vi "Multi_Point_TraverseControl.vi"(0 "Mode":T2=enum."Read traverse position", 1 "Route Checking?":bool, 3 "Traverse Name":string, 5 "RollPitchYaw":dbl[](array[numeric]) caption="Model       Roll      Pitch       Yaw (deg)" format="%#.2f", 9 "Points to plot":dbl[][](array[numeric]) format="%.2f", 11 "Work in Tunnel Coordinates?":T1, 13 "Speed Factor":dbl=1.0 min=0.1 max=5.0 format="%.2f", 14 "Backlash Compensation?":bool=TRUE) -> (4 "Position Output XYZ":dbl[](array[numeric]) format="%.2f", 15 "Error String":string)   [LabVIEW 2014]
uses:
  Anemometry/Anemometry Sub Vis/Gen Trav/Trav_mode.ctl
  Anemometry/Anemometry Sub Vis/Controls/Tunnel_Coordinates.ctl
  Anemometry/Anemometry Sub Vis/Controls/Home.ctl
  ~subVIs/GenericDriveCommand.ctl
  ADAM Client/Sub VIs/ADAM Controls/Update_scan_value.ctl
  Anemometry/Anemometry Sub Vis/Globals/Trav_pos_global.vi
  Anemometry/Anemometry Sub Vis/Globals/Preference_global.vi
  ~subVIs/DriveConfigGlobal.vi
  Anemometry/Anemometry Sub Vis/Gen Trav/Route mapping/Route_mapping_global.vi
panel:
  out "Server copy Location":path
  out "Log File":path
  out "Achieved Pos In Eng units of all channels":dbl[](array[numeric]) format="%.2f"
  out "Pulses Positon all channels":dbl[](array[numeric])
  out "Counters Reset?":bool
  # "X                Y                   Z"
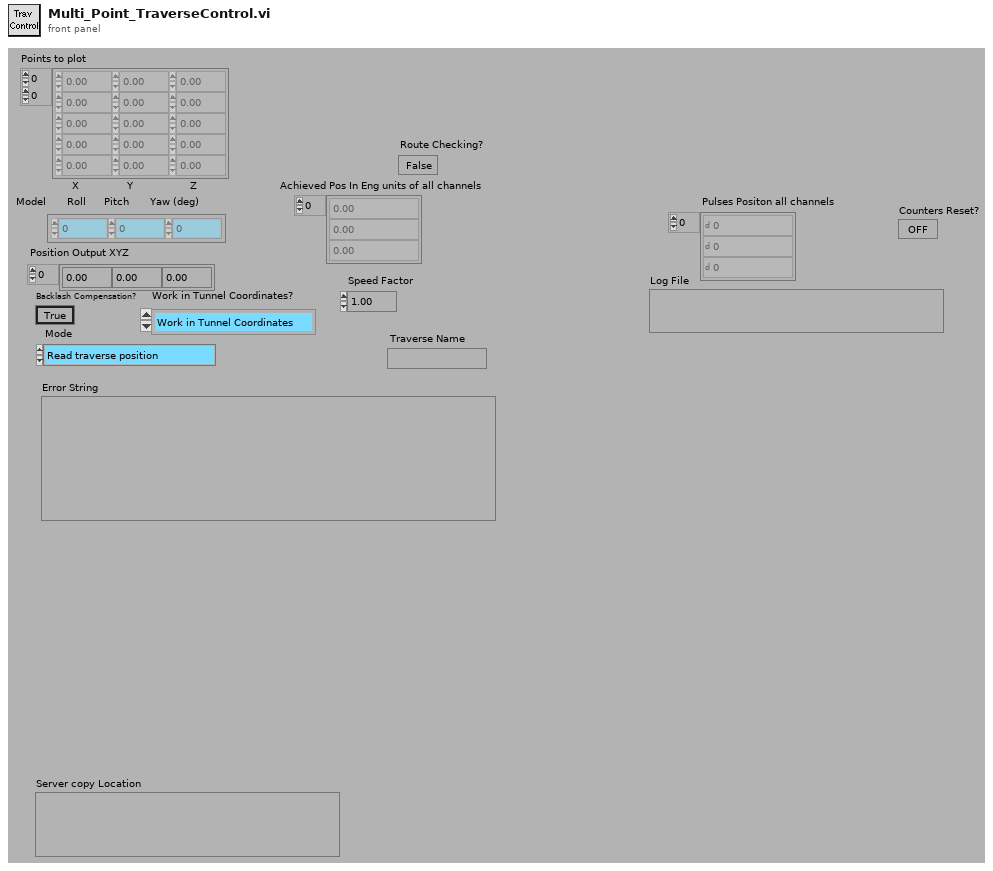
[diagram p1: front panel]
types:
  T1 = typedef "Tunnel_Coordinates.ctl" = enum16{"Work in Tunnel Coordinates", "Work in Model Coordinates"}
  T2 = typedef "Trav_mode.ctl" = enum16{"Move traverse", "Read traverse position", "Teach Position"}
  T3 = typedef "Home.ctl" = enum16{"Don't Home", "Home  +X", "Home  -X", "Home  +Y", "Home  -Y", "Home  +Z", "Home  -Z"}
  T4 = typedef "GenericDriveCommand.ctl" = string
  T5 = enum16{"To Traverse Coordinates", "To User Coordinates"}
  T6 = typedef "Update_scan_value.ctl" = cluster{"Channel Name":string, "New Value":dbl}
  T7 = typedef "AxisConfigCluster.ctl" = cluster{"Channel Properties":T8, "Static Drive Configuration":T9}
  T8 = typedef "DriveProperties.ctl" = cluster{"Channel Name":string, "Vel. Default":dbl, "Acc. Default":dbl, "Vel. Max":dbl, "Vel. Min":dbl, "Acc. Max":dbl, "Acc. Min":dbl, "Pulses/unit":dbl, "Address":u8, "Pulse Offset":i32, "Pos Tolerance":dbl, "Pulses/rev":dbl, "Backlash/Eng units":dbl, "Current Pos":dbl, "Ch Status":enum16{"Active", "Offline", "Simulate"}, "Port Name":string, "Axis Transform mode":string, "Metadata Ch Name":string, "Type":string}
  T9 = typedef "DriveStaticConfig.ctl" = cluster{"Correction Gain % (CG)":u16, "Dead Band (DB)":i32, "Dead Band Window (DW)":i32, "Encoder Resolution (ER)":i32, "Step Mode  (FSB)":u16, "Position Maintenance (FSC)":u16, "Stop on Stall (FSD)":u16, "Activate OP1 on stall (FSE)":u16, "Stop on Trigger 3 (FSF)":u16, "OP2 in Deadband (FSG)":u16, "Stall Detect (FSH)":u16, "Limit Disable (LD)":u16, "Motor Resolution (MR)":enum16{"200", "400", "1000", "2000", "4000", "5000", "10000", "12800", "18000", "20000", "21600", "25000", "25400", "25600", "36000", "50000", "278528", "425984", "507904", "614400", "655360", "819200", "1024000"}, "Limit Switch Sense (OSA)":u16, "Home Position (OSB)":u16, "Home Switch Sense (OSC)":u16, "Encoder Z for Home (OSD)":u16, "Reference edge of Home (OSH)":u16, "RS232 Echo Control (SSA)":u16, "Buffer at Limit (SSG)":u16, "Buffer at Stop (SSH)":u16, "Indexer Mode  (FSA)":u16, "Type":string, "ConfigString":string, "De Power Motor":enum16{"TRUE", "FALSE"}}
  T10 = typedef "Box_size.ctl" = cluster{"Max":dbl, "Min":dbl}[]
  T11 = typedef "Exclude_cluster.ctl" = cluster{"Sizes":T10, "Name":string, "Exclude Type":T12}
  T12 = typedef "Exclusion_type.ctl" = enum16{"Exclude completely", "Allow only vertical moves"}
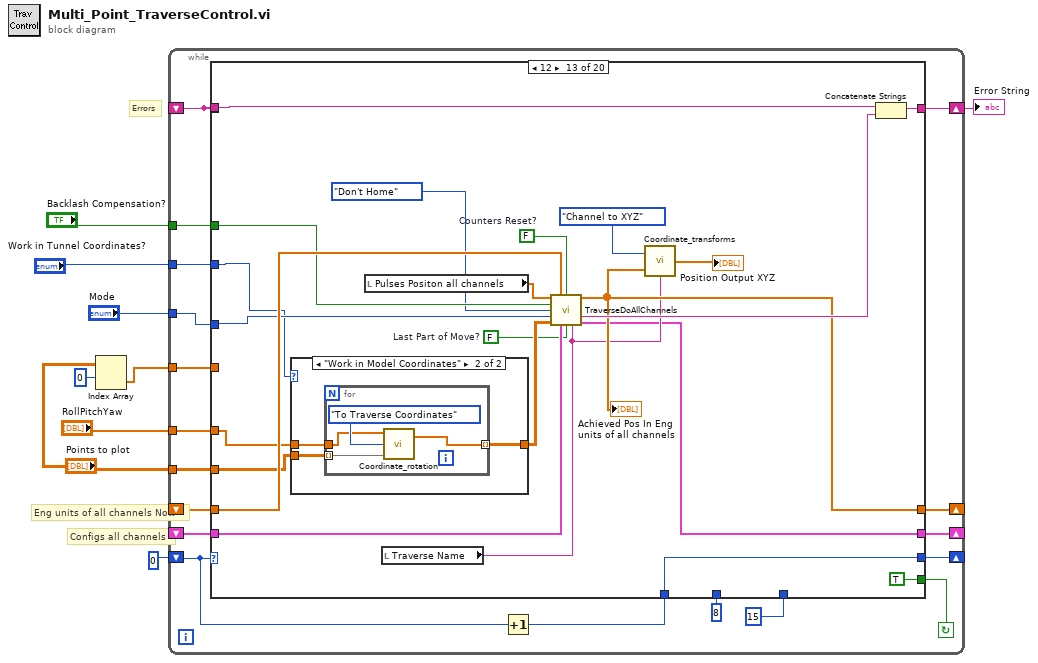
[diagram p0: block diagram]
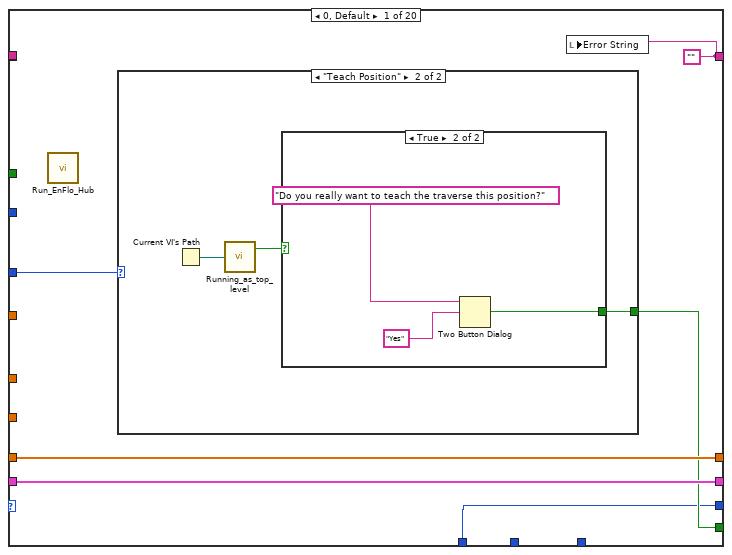
[diagram p2: hidden frame]
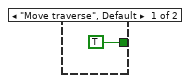
[diagram p3: hidden frame]
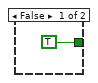
[diagram p4: hidden frame]
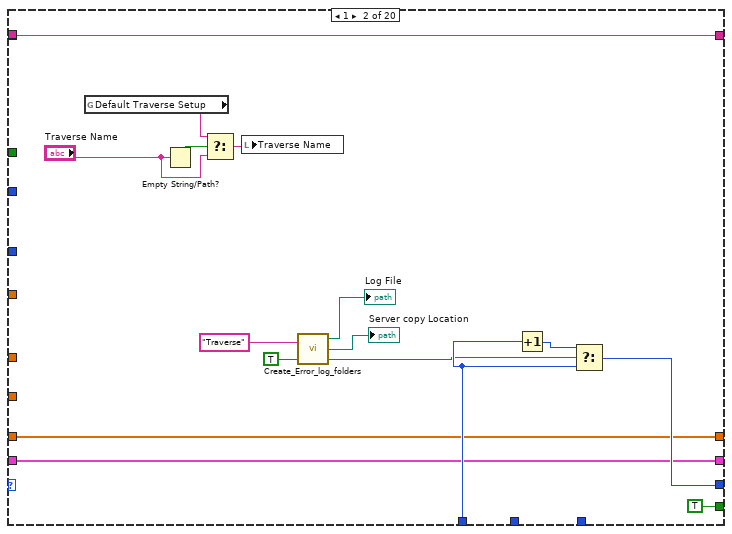
[diagram p5: hidden frame]
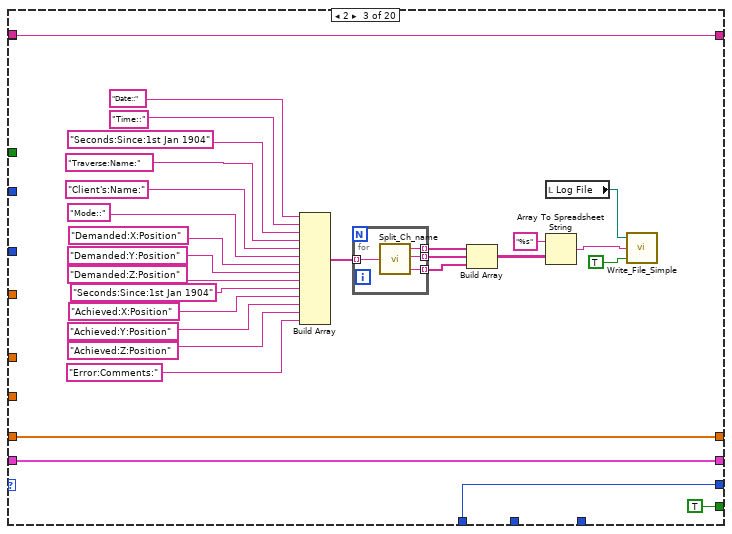
[diagram p6: hidden frame]
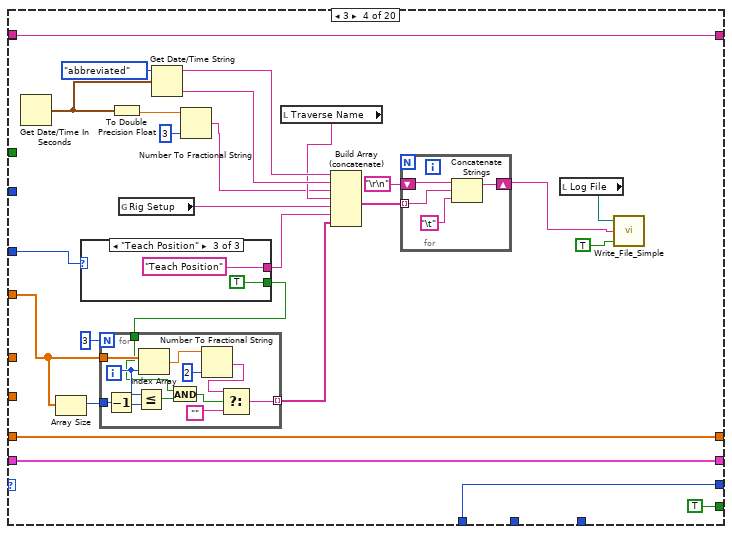
[diagram p7: hidden frame]
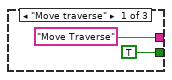
[diagram p8: hidden frame]
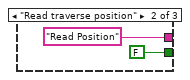
[diagram p9: hidden frame]
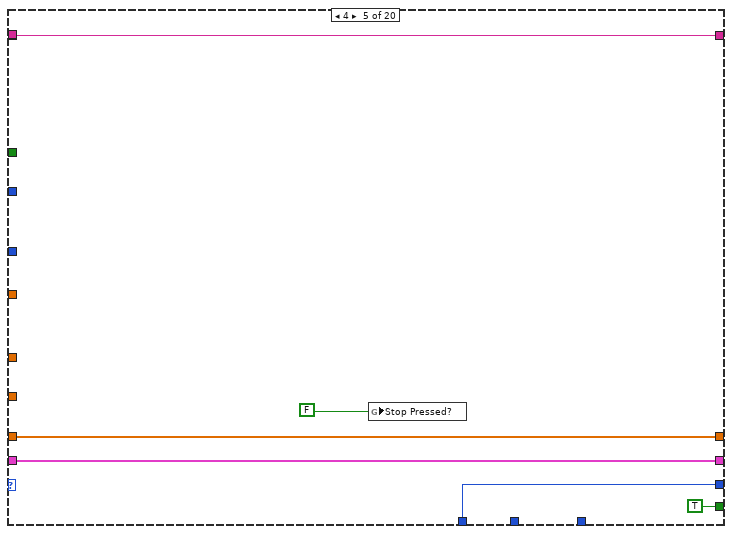
[diagram p10: hidden frame]
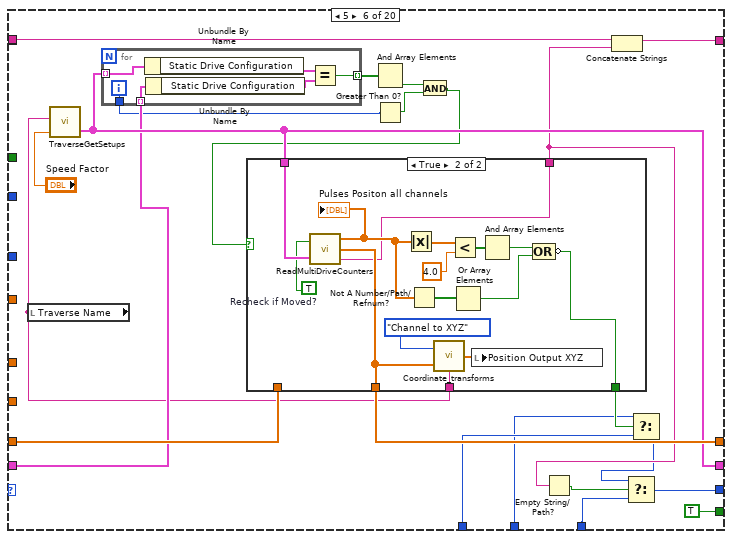
[diagram p11: hidden frame]
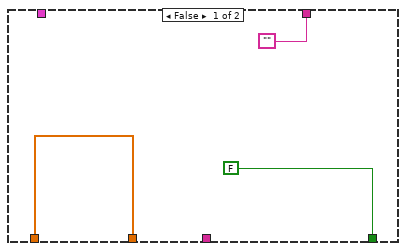
[diagram p12: hidden frame]
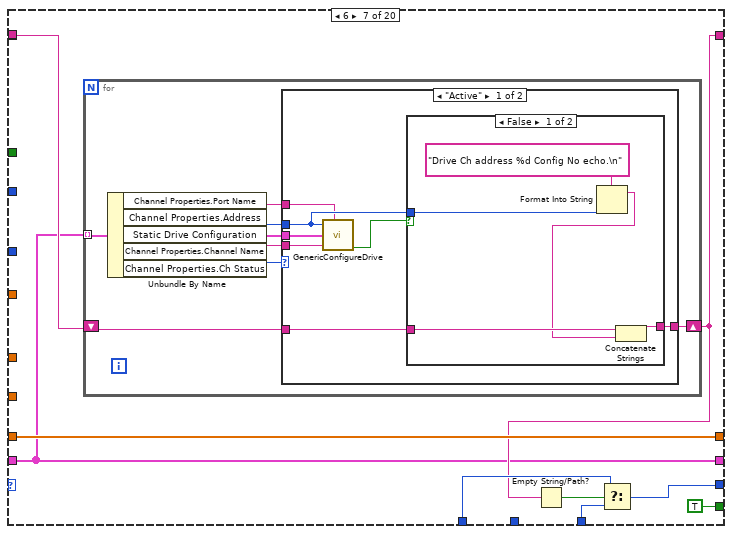
[diagram p13: hidden frame]
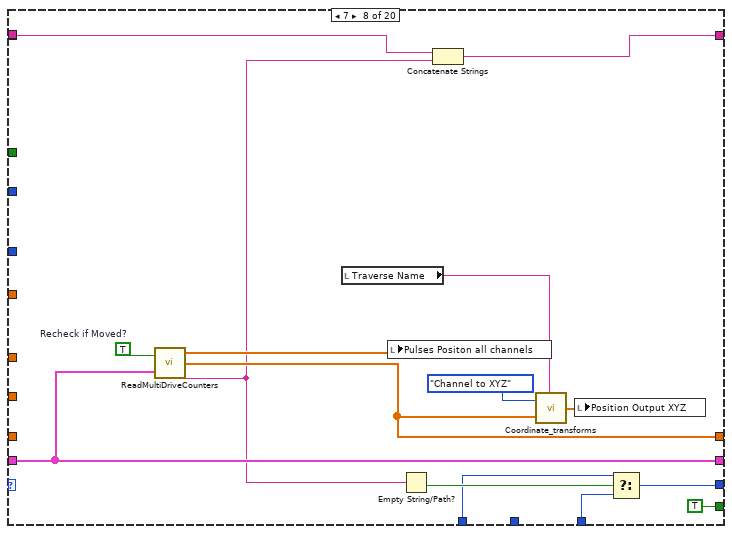
[diagram p16: hidden frame]
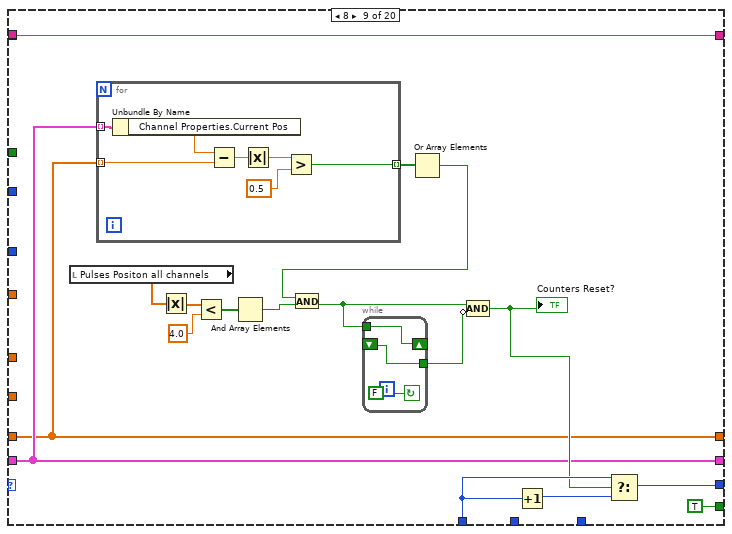
[diagram p17: hidden frame]
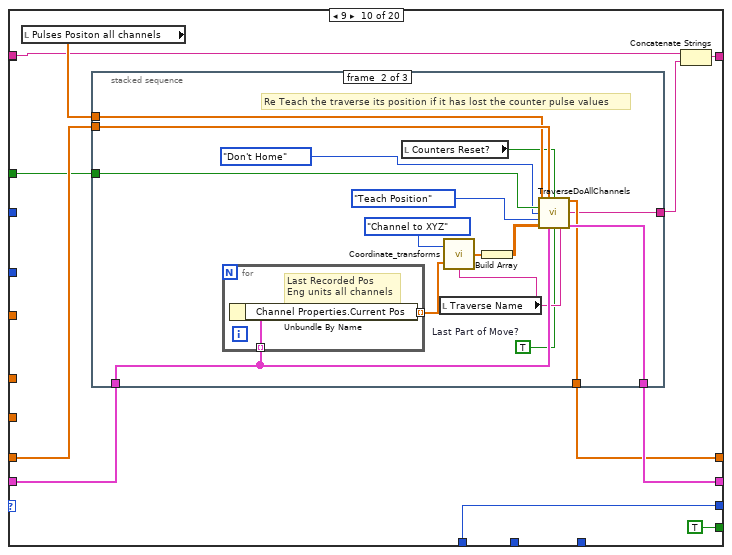
[diagram p18: hidden frame]
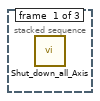
[diagram p19: hidden frame]
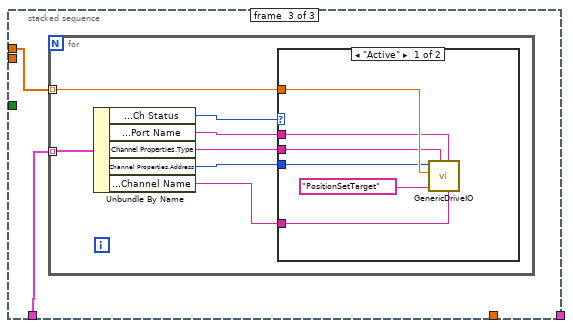
[diagram p20: hidden frame]
diagram:
  # "Errors"
  # "Eng units of all channels Now"
  # "Configs all channels"
  n1 = Index Array(array="Points to plot", index (row)=0) -> (element=w4:dbl[])  [unwired: 1 in]
  n2 = while {
    tunnel: "Backlash Compensation?" -> [w13]
    tunnel: w4 -> [w17]
    shift-left: _ -> [w14]
    shift-right: [w18] -> w7
    shift-left: _ -> [w19]
    shift-right: [w20] -> _
    shift-left: _ -> [w21]
    shift-right: [w22] -> _
    shift-left: 0 -> [w25]
    shift-right: [w23] -> _
    tunnel: "Mode" -> [w27]
    tunnel: "RollPitchYaw" -> [w12]
    tunnel: "Work in Tunnel Coordinates?" -> [w11]
    tunnel: "Points to plot" -> [w10]
    stop <- w26 continue-if-true
    n3 = Increment(x=w25) -> (x+1=w24:i32)
    n4 = case shown="12" w25 {
      tunnel: w27 -> [w33 _ _ w108 _ _ _ _ _ _ w312 _ w379 w409 _ _ _ w485 _ w541]
      tunnel: [w30 TRUE ("T button?") TRUE ("T button?") TRUE ("T button?") TRUE TRUE ("T button?") TRUE ("T button?") TRUE ("T button?") TRUE TRUE TRUE ("T button?") TRUE ("T button?") TRUE TRUE TRUE ("T button?") TRUE ("T button?") TRUE ("T button?") w487 TRUE FALSE] -> w26
      tunnel: w24 -> [w29 w56 w65 w113 w138 w162 w195 w223 w248 w264 w311 w327 w386 w411 w437 w451 w480 w484 w519 w548]
      tunnel: [w29 w54 w65 w113 w138 w145 w194 w221 w246 w264 w310 w325 w386 w410 w437 w449 w480 w483 w519 w548] -> w23
      tunnel: [w31 w51 w67 w115 w140 w160 w190 w235 w242 w273 w308 w331 w380 w408 w439 w463 w482 w490 w517 w546] -> w22
      tunnel: w21 -> [w31 w51 w67 w115 w140 w159 w190 w235 w242 w272 w308 w331 w393 w408 w439 w463 w482 w490 w517 w546]
      tunnel: [w32 w52 w66 w114 w141 w165 w198 w230 w241 w269 w307 w330 w387 w414 w438 w462 w481 w491 w520 w549] -> w20
      tunnel: w19 -> [w32 w52 w66 w114 w141 w164 w198 _ w241 w270 w307 w330 w382 w414 w438 w462 w481 w491 w520 w549]
      tunnel: [w28 w50 w63 w105 w142 w150 w191 w226 w245 w266 w313 w328 w389 w412 w435 w453 w478 w486 w513 w542] -> w18
      tunnel: w14 -> [_ w50 w63 w105 w142 w151 w192 w227 w245 w268 w313 w329 w390 w412 w435 w453 w478 w489 w515 w544]
      tunnel: w17 -> [_ _ _ w102 _ _ _ _ _ _ _ _ _ _ _ _ _ _ w511 _]
      tunnel: 15 ("f") -> [_ _ _ _ _ w146 w193 w222 _ _ _ w326 _ _ _ _ _ _ _ _]
      tunnel: 8 ("t") -> [_ _ _ _ _ w161 _ _ _ _ _ _ _ _ _ _ _ _ _ _]
      tunnel: w14 -> [_ _ _ _ _ _ _ _ _ _ _ _ _ _ _ _ _ _ _ _]
      tunnel: w13 -> [_ _ _ _ _ _ _ _ _ w263 _ _ w381 _ _ _ _ _ _ _]
      tunnel: w12 -> [_ _ _ _ _ _ _ _ _ _ _ w332 w377 _ _ _ _ _ w512 w539]
      tunnel: w11 -> [_ _ _ _ _ _ _ _ _ _ _ _ w376 _ _ _ _ _ w509 w537]
      tunnel: w10 -> [_ _ _ _ _ _ _ _ _ _ _ w333 w378 _ _ _ _ _ _ _]
      frame 0, Default {
        w28 = ""
        n5 = call "Run_EnFlo_Hub.vi"() -> ()  [unwired: 8 out]
        n6 = case shown="\"Teach Position\"" w33 {
          tunnel: [TRUE ("T button?") w35] -> w30
          frame "Move traverse", Default {
          }
          frame "Teach Position" {
            n7 = Current VI's Path() -> (path=w37:path)
            n8 = call "Running_as_top_level.vi"("Vi path name"=w37) -> ("Top Level"=w36:bool)  [unwired: 1 out]
            n9 = case shown="True" w36 {
              tunnel: [TRUE ("T button?") w39] -> w35
              frame False {
              }
              frame True {
                n10 = Two Button Dialog(message="Do you really want to teach the traverse this position?", 2:"Yes" ("T button name (\"OK\")")) -> (T button?=w39:bool)  [unwired: 1 out]
              }
            }
          }
        }
        n11 = local write "Error String"(w28) -> ()
      }
      frame 1 {
        n12 = global read "Trav_pos_global.vi" "Default Traverse Setup"() -> (w47:string)
        n13 = Empty String/Path?(string/path="Traverse Name") -> (empty?=w45:bool)
        n14 = Select(t=w47, s=w45, f="Traverse Name") -> (s? t:f=w44:string)
        n15 = local write "Traverse Name"(w44) -> ()
        n16 = call "Create_Error_log_folders.vi"("Per Day Log File?"=TRUE, "Log Filename"="Traverse" ("Input Element")) -> ("exists?"=w48:bool, "Server copy Location"=→"Server copy Location":path, "Local Log File"=→"Log File":path)  [unwired: 1 in]
        n17 = Increment(x=w56) -> (x+1=w55:i32)
        n18 = Select(t=w55, s=w48, f=w56) -> (s? t:f=w54:i32)
      }
      frame 2 {
        n19 = Build Array("Date::", "Time::", "Seconds:Since:1st Jan 1904", "Traverse:Name:", "Client's:Name:", "Mode::", "Demanded:X:Position", "Demanded:Y:Position", "Demanded:Z:Position", "Seconds:Since:1st Jan 1904", "Achieved:X:Position", "Achieved:Y:Position", "Achieved:Z:Position", "Error:Comments:") -> (w70:string[])
        n20 = for {
          tunnel: w70 -> [w89] mode=indexing
          tunnel: [w88] -> w71 mode=indexing
          tunnel: [w87] -> w72 mode=indexing
          tunnel: [w86] -> w73 mode=indexing
          n21 = call "Split_Ch_name.vi"("Ch name"=w89) -> ("Top level"=w88:string, "Middle"=w87:string, "Low level"=w86:string)
        }
        n22 = Build Array(w71, w72, w73) -> (w68:string[][])
        n23 = local read "Log File"() -> (w59:path)
        n24 = Array To Spreadsheet String(array=w68, 3:"%s" ("format string")) -> (spreadsheet string=w60:string)  [unwired: 1 out]
        n25 = call "Write_File_Simple.vi"("append to file? (new file:F)"=TRUE, "character string"=w60, "file path"=w59) -> ()  [unwired: 2 out]
      }
      frame 3 {
        n26 = Get Date/Time In Seconds() -> (seconds since 1Jan1904=w94:timestamp)
        n27 = Array Size(array=w102) -> (size(s)=w103:i32)
        n28 = case shown="\"Teach Position\"" w108 {
          tunnel: ["Move Traverse" "Read Position" "Teach Position"] -> w109
          tunnel: [TRUE FALSE TRUE] -> w99
          frame "Move traverse" {
          }
          frame "Read traverse position" {
          }
          frame "Teach Position" {
          }
        }
        n29 = for {
          N: 3 -> [_]
          tunnel: w102 -> [w127]
          tunnel: w103 -> [w124]
          tunnel: [w120] -> w100 mode=indexing
          tunnel: w99 -> [w116]
          i -> [w122]
          n30 = Decrement(x=w124) -> (x-1=w123:i32)
          n31 = Less Or Equal?(x=w122, y=w123) -> (x <= y?=w118:bool)
          n32 = Index Array(array=w127, index=w122) -> (element=w126:dbl)
          n33 = And(x=w116, y=w118) -> (x .and. y?=w117:bool)
          n34 = Number To Fractional String(number=w126, precision (6)=i16 2) -> (F-format string=w121:string)  [unwired: 2 out]
          n35 = Select(t=w121, s=w117, f="") -> (s? t:f=w120:string)
        }
        n36 = To Double Precision Float(number=w94) -> (double precision float=w93:dbl)
        n37 = global read "Preference_global.vi" "Rig Setup"() -> (w90:string)
        n38 = Get Date/Time String(date format (0)=enum16{"short", "long", "abbreviated"}."abbreviated", seconds (now)=w94) -> (date string=w111:string, time string=w110:string)  [unwired: 1 out]
        n39 = Number To Fractional String(number=w93, precision (6)=i16 3) -> (F-format string=w91:string)  [unwired: 2 out]
        n40 = local read "Traverse Name"() -> (w95:string)
        n41 = Build Array (concatenate)(w111, w110, w91, w95, w90, w109, w100) -> (w106:string[])
        n42 = for {
          shift-right: [w130] -> w96
          shift-left: "\r\n" -> [w131]
          tunnel: w106 -> [w129] mode=indexing
          n43 = Concatenate Strings(w131, w129, "\t") -> (w130:string)
        }
        n44 = local read "Log File"() -> (w97:path)
        n45 = call "Write_File_Simple.vi"("append to file? (new file:F)"=TRUE, "character string"=w96, "file path"=w97) -> ()  [unwired: 2 out]
      }
      frame 4 {
        n46 = global write "DriveConfigGlobal.vi" "Stop Pressed?"(FALSE) -> ()
      }
      frame 5 {
        n47 = local read "Traverse Name"() -> (w153:string)
        n48 = call "TraverseGetSetups.vi"("Speed Factor"="Speed Factor", "Traverse Name"=w153) -> ("Matched Configurations"=w160:T7[])  [unwired: 2 in]
        n49 = for {
          tunnel: w160 -> [w171] mode=indexing
          tunnel: w159 -> [w170] mode=indexing
          tunnel: [w167] -> w158 mode=indexing
          tunnel: [w166] -> w157
          i -> [w166]
          n50 = Unbundle By Name(w171) -> ("Static Drive Configuration"=w169:T9)
          n51 = Unbundle By Name(w170) -> ("Static Drive Configuration"=w168:T9)
          n52 = Equal?(x=w169, y=w168) -> (x = y?=w167:bool)
        }
        n53 = And Array Elements(Boolean array=w158) -> (logical AND=w155:bool)
        n54 = Greater Than 0?(x=w157) -> (x > 0?=w156:bool)
        n55 = And(x=w155, y=w156) -> (x .and. y?=w154:bool)
        n56 = case shown="True" w154 {
          tunnel: w160 -> [_ w189]
          tunnel: [w174 w179] -> w165
          tunnel: w164 -> [w174 _]
          tunnel: [FALSE w181] -> w163
          tunnel: w153 -> [_ w177]
          tunnel: ["" w175] -> w149
          frame False {
          }
          frame True {
            w176 = TRUE  # Recheck if Moved?
            n57 = call "ReadMultiDriveCounters.vi"("Recheck if Moved?"=w176, "Matched Configurations"=w189) -> ("Pulses"=w184:dbl[], "Eng units"=w179:dbl[], "Error String"=w175:string)
            "Pulses Positon all channels" <- w184
            n58 = Absolute Value(x=w184) -> (abs(x)=w188:dbl[])
            n59 = Not A Number/Path/Refnum?(number/path/refnum=w184) -> (NaN/Path/Refnum?=w183:bool[])
            n60 = call "Coordinate_transforms.vi"("Traverse Name"=w177, "Input"=w179, "Mode"=enum16{"XYZ to Channel", "Channel to XYZ"}."Channel to XYZ") -> ("Output"=w178:dbl[])
            n61 = Less?(x=w188, y=4.0 ("Achieved Position")) -> (x < y?=w186:bool[])
            n62 = Or Array Elements(Boolean array=w183) -> (logical OR=w182:bool)
            n63 = local write "Position Output XYZ"(w178) -> ()
            n64 = And Array Elements(Boolean array=w186) -> (logical AND=w185:bool)
            n65 = Compound Arithmetic op=OR(w185, w182) -> (invert w181:bool)
          }
        }
        n66 = Empty String/Path?(string/path=w149) -> (empty?=w148:bool)
        n67 = Concatenate Strings(w151, w149) -> (w150:string)
        n68 = Select(t=w161, s=w163, f=w162) -> (s? t:f=w147:i32)
        n69 = Select(t=w147, s=w148, f=w146) -> (s? t:f=w145:i32)
      }
      frame 6 {
        n70 = for {
          tunnel: w190 -> [w206] mode=indexing
          shift-right: [w199] -> w191
          shift-left: w192 -> [w200]
          n71 = Unbundle By Name(w206) -> ("Channel Properties.Port Name"=w201:string, "Channel Properties.Address"=w205:u8, "Static Drive Configuration"=w204:T9, "Channel Properties.Channel Name"=w203:string, "Channel Properties.Ch Status"=w202:enum16{"Active", "Offline", "Simulate"})
          n72 = case shown="\"Active\"" w202 {
            tunnel: w205 -> [w211 _]
            tunnel: w204 -> [w213 _]
            tunnel: w203 -> [w212 _]
            tunnel: w201 -> [w210 _]
            tunnel: w200 -> [w208 w220]
            tunnel: [w207 w220] -> w199
            frame "Active" {
              n73 = call "GenericConfigureDrive.vi"("Address"=w211, "Port Name"=w210, "Static Drive Configuration"=w213, "Channel Name"=w212) -> ("Good Echo"=w209:bool)  [unwired: 4 out]
              n74 = case shown="False" w209 {
                tunnel: w211 -> [w218 _]
                tunnel: w208 -> [w216 w219]
                tunnel: [w215 w219] -> w207
                frame False {
                  n75 = Format Into String(format string="Drive Ch address %d Config No echo.\n" ("Format String"), w218) -> (resulting string=w214:string)  [unwired: 2 in, 1 out]
                  n76 = Concatenate Strings(w216, w214) -> (w215:string)
                }
                frame True {
                }
              }
            }
            frame "Offline", Default {
            }
          }
        }
        n77 = Empty String/Path?(string/path=w191) -> (empty?=w196:bool)
        n78 = Select(t=w195, s=w196, f=w193) -> (s? t:f=w194:i32)
      }
      frame 7 {
        w228 = TRUE  # Recheck if Moved?
        n79 = call "ReadMultiDriveCounters.vi"("Recheck if Moved?"=w228, "Matched Configurations"=w235) -> ("Pulses"=w233:dbl[], "Eng units"=w230:dbl[], "Error String"=w224:string)
        n80 = local read "Traverse Name"() -> (w229:string)
        n81 = local write "Pulses Positon all channels"(w233) -> ()
        n82 = Empty String/Path?(string/path=w224) -> (empty?=w225:bool)
        n83 = Concatenate Strings(w227, w224) -> (w226:string)
        n84 = call "Coordinate_transforms.vi"("Traverse Name"=w229, "Input"=w230, "Mode"=enum16{"XYZ to Channel", "Channel to XYZ"}."Channel to XYZ") -> ("Output"=w231:dbl[])
        n85 = local write "Position Output XYZ"(w231) -> ()
        n86 = Select(t=w223, s=w225, f=w222) -> (s? t:f=w221:i32)
      }
      frame 8 {
        n87 = local read "Pulses Positon all channels"() -> (w236:dbl[])
        n88 = for {
          tunnel: w242 -> [w262] mode=indexing
          tunnel: w241 -> [w260] mode=indexing
          tunnel: [w256] -> w239 mode=indexing
          n89 = Unbundle By Name(w262) -> ("Channel Properties.Current Pos"=w261:dbl)
          n90 = Subtract(x=w261, y=w260) -> (x-y=w259:dbl)
          n91 = Absolute Value(x=w259) -> (abs(x)=w258:dbl)
          n92 = Greater?(x=w258, y=0.5) -> (0:w256:bool)
        }
        n93 = Absolute Value(x=w236) -> (abs(x)=w252:dbl[])
        n94 = Less?(x=w252, y=4.0 ("Achieved Position")) -> (x < y?=w250:bool[])
        n95 = And Array Elements(Boolean array=w250) -> (logical AND=w240:bool)
        n96 = Or Array Elements(Boolean array=w239) -> (logical OR=w238:bool)
        n97 = And(x=w238, y=w240) -> (x .and. y?=w237:bool)
        n98 = while {
          tunnel: [w254] -> w244
          tunnel: w237 -> [w255]
          shift-left: _ -> [w254]
          shift-right: [w255] -> _
          stop <- FALSE continue-if-true
        }
        n99 = Compound Arithmetic op=AND(w237, invert w244) -> (w243:bool)
        "Counters Reset?" <- w243
        n100 = Increment(x=w248) -> (x+1=w247:i32)
        n101 = Select(t=w248, s=w243, f=w247) -> (s? t:f=w246:i32)
      }
      frame 9 {
        n102 = local read "Pulses Positon all channels"() -> (w271:dbl[])
        n103 = stacked-sequence {
          tunnel: w271 -> [_ w281 w292]
          tunnel: [_ w289 _] -> w273
          tunnel: w270 -> [_ w288 _]
          tunnel: [_ w287 _] -> w269
          tunnel: w272 -> [_ w283 w293]
          tunnel: [_ w286 _] -> w267
          tunnel: w263 -> [_ w277 _]
          frame #0 {
            n104 = call "Shut_down_all_Axis.vi"() -> ()  [unwired: 1 out]
          }
          frame #1 {
            w275 = TRUE  # Last Part of Move?
            # "Re Teach the traverse its position if it has lost the counter pulse values"
            n105 = for {
              tunnel: [w291] -> w282 mode=indexing
              tunnel: w283 -> [w290] mode=indexing
              # "Last Recorded Pos\nEng units all channels"
              n106 = Unbundle By Name(w290) -> ("Channel Properties.Current Pos"=w291:dbl)
            }
            n107 = local read "Counters Reset?"() -> (w279:bool)
            n108 = local read "Traverse Name"() -> (w278:string)
            n109 = call "Coordinate_transforms.vi"("Traverse Name"=w278, "Input"=w282, "Mode"=enum16{"XYZ to Channel", "Channel to XYZ"}."Channel to XYZ") -> ("Output"=w284:dbl[])
            n110 = Build Array(w284) -> (w276:dbl[][])
            n111 = call "TraverseDoAllChannels.vi"("Current Pulses positions for all channels"=w281, "Current Pos In Eng units of all channels"=w288, "Counters Reset?"=w279, "Backlash Compensation?"=w277, "Home"=Home."Don't Home", "Mode"=Trav_mode."Teach Position", "Position Steps"=w276, "Matched Configurations all Channels In"=w283, "Last Part of Move?"=w275, "Traverse Name"=w278) -> ("Achieved Pos In Eng units of all channels"=w287:dbl[], "Error String"=w286:string, "Matched Configurations Out"=w289:T7[])  [unwired: 2 in, 1 out]
          }
          frame #2 {
            n112 = for {
              tunnel: w293 -> [w300] mode=indexing
              tunnel: w292 -> [w299] mode=indexing
              n113 = Unbundle By Name(w300) -> ("Channel Properties.Ch Status"=w298:enum16{"Active", "Offline", "Simulate"}, "Channel Properties.Port Name"=w297:string, "Channel Properties.Type"=w296:string, "Channel Properties.Address"=w295:u8, "Channel Properties.Channel Name"=w294:string)
              n114 = case shown="\"Active\"" w298 {
                tunnel: w299 -> [w306 _]
                tunnel: w297 -> [w305 _]
                tunnel: w296 -> [w304 _]
                tunnel: w295 -> [w303 _]
                tunnel: w294 -> [w302 _]
                frame "Active" {
                  n115 = call "GenericDriveIO.vi"("GenericDriveCommand"=T4 "PositionSetTarget", "Channel Name"=w302, "Numeric Value"=w306, "Address"=w303, "Type"=w304, "Port Name"=w305) -> ()  [unwired: 1 in, 5 out]
                }
                frame "Offline", Default {
                }
              }
            }
          }
        }
        n116 = Concatenate Strings(w268, w267) -> (w266:string)
      }
      frame 10 {
        n117 = case shown="\"Move traverse\"" w312 {
          tunnel: w311 -> [w314 w321]
          tunnel: [w316 w320] -> w310
          frame "Move traverse" {
            n118 = Increment(x=w314) -> (x+1=w315:i32)
            n119 = case shown="True" "Route Checking?" {
              tunnel: [w318 w319] -> w316
              tunnel: w315 -> [w318 _]
              tunnel: w314 -> [_ w319]
              frame False {
              }
              frame True {
              }
            }
          }
          frame "Read traverse position", Default {
            n120 = Increment(x=w321) -> (x+1=w320:i32)
          }
        }
      }
      frame 11 {
        w342 = 0.1  # Reduce by
        n121 = global read "Route_mapping_global.vi" "Probe Volume"() -> (w343:T10)
        n122 = local read "Traverse Name"() -> (w324:string)
        n123 = for {
          tunnel: w343 -> [w372] mode=indexing
          tunnel: [w371] -> w344 mode=indexing
          tunnel: w342 -> [w366]
          n124 = Unbundle By Name(w372) -> ("Max"=w370:dbl, "Min"=w368:dbl)
          n125 = Subtract(x=w370, y=w366) -> (x-y=w369:dbl)
          n126 = Add(x=w366, y=w368) -> (x+y=w367:dbl)
          n127 = Bundle By Name(cluster=w372, "Max"=w369, "Min"=w367) -> (w371:cluster{"Max":dbl, "Min":dbl})
        }
        n128 = global read "Route_mapping_global.vi" "Probe Support"() -> (w322:T10)
        n129 = global read "Route_mapping_global.vi" "Entire Space"() -> (w341:T10)
        n130 = global read "Route_mapping_global.vi" "Exclude Array"() -> (w340:T11[])
        n131 = call "Coordinate_transforms.vi"("Traverse Name"=w324, "Input"=w330, "Mode"=enum16{"XYZ to Channel", "Channel to XYZ"}."Channel to XYZ") -> ("Output"=w338:dbl[])
        n132 = Array Size(array=w333) -> (size(s)=w345:i32[])
        n133 = Index Array(array=w345, index=0) -> (element=w347:i32)
        n134 = call "Coordinate_rotation.vi"("Model       Roll      Pitch       Yaw (deg)"=w332, "Input Position"=w338, "Mode"=T5."To User Coordinates") -> ("Output Position"=w335:dbl[])  [unwired: 2 in, 1 out]
        n135 = Decrement(x=w347) -> (x-1=w348:i32)
        n136 = while {
          tunnel: w335 -> [w364]
          tunnel: w333 -> [w362] mode=indexing
          tunnel: w324 -> [w361]
          tunnel: w332 -> [w359]
          tunnel: [w355] -> w339
          tunnel: w340 -> [w358]
          tunnel: w341 -> [w357]
          tunnel: w344 -> [w356]
          tunnel: w348 -> [w353]
          tunnel: w322 -> [w349]
          i -> [w354]
          stop <- w350 continue-if-true
          w360 = FALSE  # Full Check
          n137 = Less?(x=w354, y=w353) -> (x < y?=w351:bool)
          n138 = call "Coordinate_rotation.vi"("Model       Roll      Pitch       Yaw (deg)"=w359, "Input Position"=w362, "Mode"=T5."To User Coordinates") -> ("Output Position"=w363:dbl[])  [unwired: 2 in, 1 out]
          n139 = call "Check_Traverse_move.vi"("Current position"=w364, "Traverse Name"=w361, "Full Check"=w360, "New Position"=w363, "Model       Roll      Pitch       Yaw (deg)"=w359, "Probe Volume"=w356, "Entire Space"=w357, "Exclude Array"=w358, "Probe Support"=w349) -> ("Error Comments"=w355:string)  [unwired: 6 out]
          n140 = Empty String/Path?(string/path=w355) -> (empty?=w352:bool)
          n141 = And(x=w352, y=w351) -> (x .and. y?=w350:bool)
        }
        n142 = Empty String/Path?(string/path=w339) -> (empty?=w336:bool)
        n143 = Select(t=w327, s=w336, f=w326) -> (s? t:f=w325:i32)
        n144 = Concatenate Strings(w329, w339) -> (w328:string)
      }
      frame 12 {
        w374 = FALSE  # Last Part of Move?
        w384 = FALSE  # Counters Reset?
        n145 = case shown="\"Work in Model Coordinates\"" w376 {
          tunnel: w377 -> [_ w398]
          tunnel: w378 -> [w395 w397]
          tunnel: [w395 w396] -> w375
          frame "Work in Tunnel Coordinates" {
          }
          frame "Work in Model Coordinates" {
            n146 = for {
              tunnel: w397 -> [w401] mode=indexing
              tunnel: [w400] -> w396 mode=indexing
              tunnel: w398 -> [w399]
              n147 = call "Coordinate_rotation.vi"("Model       Roll      Pitch       Yaw (deg)"=w399, "Input Position"=w401, "Mode"=T5."To Traverse Coordinates") -> ("Output Position"=w400:dbl[])  [unwired: 2 in, 1 out]
            }
          }
        }
        n148 = local read "Pulses Positon all channels"() -> (w394:dbl[])
        n149 = local read "Traverse Name"() -> (w383:string)
        n150 = call "TraverseDoAllChannels.vi"("Current Pulses positions for all channels"=w394, "Current Pos In Eng units of all channels"=w382, "Counters Reset?"=w384, "Backlash Compensation?"=w381, "Home"=Home."Don't Home", "Mode"=w379, "Position Steps"=w375, "Matched Configurations all Channels In"=w393, "Last Part of Move?"=w374, "Traverse Name"=w383) -> ("Achieved Pos In Eng units of all channels"=w387:dbl[], "Error String"=w388:string, "Matched Configurations Out"=w380:T7[])  [unwired: 2 in, 1 out]
        "Achieved Pos In Eng units of all channels" <- w387
        n151 = call "Coordinate_transforms.vi"("Traverse Name"=w383, "Input"=w387, "Mode"=enum16{"XYZ to Channel", "Channel to XYZ"}."Channel to XYZ") -> ("Output"=→"Position Output XYZ":dbl[])
        n152 = Concatenate Strings(w390, w388) -> (w389:string)
      }
      frame 13 {
        n153 = local read "Position Output XYZ"() -> (w406:dbl[])
        n154 = case shown="\"Read traverse position\"" w409 {
          tunnel: w406 -> [_ _ _]
          frame "Move traverse" {
          }
          frame "Read traverse position" {
          }
          frame "Teach Position" {
            n155 = local write "Mode"(Trav_mode."Teach Position" ("Mode")) -> ()
          }
        }
        n156 = for {
          tunnel: w408 -> [w426] mode=indexing
          tunnel: T6 {"Channel Name"="", "New Value"=0.0} ("Update Scan Value Cluster") -> [w425]
          tunnel: w406 -> [w423] mode=indexing
          shift-right: [w421] -> w404
          shift-left: T6[] [] -> [w422]
          n157 = Unbundle By Name(w426) -> ("Channel Properties.Metadata Ch Name"=w424:string, "Channel Properties.Ch Status"=w420:enum16{"Active", "Offline", "Simulate"})
          n158 = Equal?(x=w420, y=enum16{"Active", "Offline", "Simulate"}."Active" ("Channel Properties.Ch Status")) -> (x = y?=w418:bool)
          n159 = Empty String/Path?(string/path=w424) -> (empty?=w417:bool)
          n160 = Compound Arithmetic op=AND(invert w417, w418) -> (w416:bool)
          n161 = case shown="True" w416 {
            tunnel: w425 -> [_ w433]
            tunnel: w424 -> [_ w432]
            tunnel: w423 -> [_ w431]
            tunnel: w422 -> [w427 w429]
            tunnel: [w427 w428] -> w421
            frame False {
            }
            frame True {
              n162 = Bundle By Name(cluster=w433, "Channel Name"=w432, "New Value"=w431) -> (w430:T6)
              n163 = Build Array (concatenate)(w429, w430) -> (w428:T6[])
            }
          }
        }
        n164 = global write "DriveConfigGlobal.vi" "Run Emergency stop loop"(FALSE ("Run Emergency stop loop")) -> ()
        n165 = Increment(x=w411) -> (x+1=w410:i32)
        n166 = call "Update_Current_Value_client.vi"("Don't Bother with check?"=FALSE, "Update array in"=w404) -> ()
      }
      frame 14 {
      }
      frame 15 {
        n167 = local read "Position Output XYZ"() -> (w457:dbl[])
        n168 = Array Size(array=w457) -> (size(s)=w456:i32)
        n169 = Get Date/Time In Seconds() -> (seconds since 1Jan1904=w448:timestamp)
        n170 = for {
          N: 3 -> [_]
          tunnel: w457 -> [w477]
          tunnel: w456 -> [w474]
          tunnel: [w469] -> w455 mode=indexing
          i -> [w472]
          n171 = Decrement(x=w474) -> (x-1=w473:i32)
          n172 = Less Or Equal?(x=w472, y=w473) -> (x <= y?=w471:bool)
          n173 = Index Array(array=w477, index=w472) -> (element=w476:dbl)
          n174 = Number To Fractional String(number=w476, precision (6)=i16 2) -> (F-format string=w470:string)  [unwired: 2 out]
          n175 = Select(t=w470, s=w471, f="") -> (s? t:f=w469:string)
        }
        n176 = To Double Precision Float(number=w448) -> (double precision float=w441:dbl)
        n177 = Number To Fractional String(number=w441, precision (6)=i16 3) -> (F-format string=w440:string)  [unwired: 2 out]
        n178 = call "Remove_unprintable_Char.vi"("Input String"=w453) -> ("Output String"=w454:string)
        n179 = Build Array (concatenate)(w440, w455, w454) -> (w459:string[])
        n180 = local read "Route Checking?"() -> (w452:bool)
        n181 = for {
          shift-right: [w466] -> w445
          shift-left: "" -> [w467]
          tunnel: w459 -> [w465] mode=indexing
          n182 = Concatenate Strings(w467, w465, "\t") -> (w466:string)
        }
        n183 = Increment(x=w451) -> (x+1=w450:i32)
        n184 = local read "Log File"() -> (w446:path)
        n185 = local read "Server copy Location"() -> (w443:path)
        n186 = Select(t=w450, s=w452, f=w451) -> (s? t:f=w449:i32)
        n187 = call "Write_File_Simple.vi"("append to file? (new file:F)"=TRUE, "character string"=w445, "file path"=w446) -> ("file path Out"=w444:path)  [unwired: 1 out]
        n188 = call "Updated_File_Copy.vi"("Target Path"=w443, "Source Path"=w444) -> ()  [unwired: 2 out]
      }
      frame 16 {
      }
      frame 17 {
        n189 = local read "Position Output XYZ"() -> (w492:dbl[])
        n190 = local read "Counters Reset?"() -> (w493:bool)
        n191 = Index Array(array=w492, index=2) -> (element=w498:dbl)
        n192 = Index Array(array=w492, index=0) -> (element=w500:dbl)
        n193 = Index Array(array=w492, index=1) -> (element=w499:dbl)
        n194 = Format Into String(format string="X= %.2f\tY= %.2f\tZ= %.2f" ("Format String"), w500, w499, w498) -> (resulting string=w501:string)  [unwired: 2 in, 1 out]
        n195 = case shown="\"Read traverse position\"" w485 {
          tunnel: w484 -> [w505 w507]
          tunnel: [w505 w506] -> w483
          frame "Move traverse", Default {
          }
          frame "Read traverse position" {
            n196 = Increment(x=w507) -> (x+1=w506:i32)
          }
        }
        n197 = Select(t="\nThe traverse was probably powered down since the last move. Its position has now been retaught and now all should be well.", s=w493, f="") -> (s? t:f=w494:string)
        n198 = call "Write_out_serial_log.vi"("Header message"=w501) -> ()
        n199 = Concatenate Strings(w489, w494) -> (w486:string)
        n200 = Empty String/Path?(string/path=w486) -> (empty?=w488:bool)
        n201 = Not(x=w488) -> (.not. x?=w487:bool)
      }
      frame 18 {
        # "Add demanded position"
        n202 = case shown="\"Work in Model Coordinates\"" w509 {
          tunnel: w512 -> [_ w527]
          tunnel: w511 -> [w522 w526]
          tunnel: [w522 w524] -> w510
          tunnel: [" (Tunnel Coordinates)" " (Model Coordinates)"] -> w508
          frame "Work in Tunnel Coordinates" {
          }
          frame "Work in Model Coordinates" {
            n203 = call "Coordinate_rotation.vi"("Model       Roll      Pitch       Yaw (deg)"=w527, "Input Position"=w526, "Mode"=T5."To User Coordinates") -> ("Output Position"=w524:dbl[])  [unwired: 2 in, 1 out]
          }
        }
        n204 = for {
          tunnel: w517 -> [w535] mode=indexing
          shift-right: [w530] -> w514
          shift-left: "\nDem Pos " -> [w533]
          tunnel: w510 -> [w528] mode=indexing
          n205 = Unbundle By Name(w535) -> ("Channel Properties.Channel Name"=w534:string)
          n206 = call "Split_Ch_name.vi"("Ch name"=w534) -> ("Low level"=w532:string)  [unwired: 2 out]
          n207 = Format Into String(format string="%s=%.1f, " ("Format String"), w532, w528) -> (resulting string=w529:string)  [unwired: 2 in, 1 out]
          n208 = Concatenate Strings(w533, w529) -> (w530:string)
        }
        n209 = Concatenate Strings(w515, w514, w508) -> (w513:string)
      }
      frame 19 {
        # "Add Achieved Position"
        n210 = local read "Position Output XYZ"() -> (w536:dbl[])
        n211 = case shown="\"Work in Model Coordinates\"" w537 {
          tunnel: w539 -> [_ w553]
          tunnel: [w550 w552] -> w538
          tunnel: w536 -> [w550 w551]
          frame "Work in Tunnel Coordinates" {
          }
          frame "Work in Model Coordinates" {
            n212 = call "Coordinate_rotation.vi"("Model       Roll      Pitch       Yaw (deg)"=w553, "Input Position"=w551, "Mode"=T5."To User Coordinates") -> ("Output Position"=w552:dbl[])  [unwired: 2 in, 1 out]
          }
        }
        n213 = for {
          tunnel: w546 -> [w565] mode=indexing
          shift-right: [w560] -> w543
          shift-left: "\nAchieved Pos " -> [w563]
          tunnel: w538 -> [w558] mode=indexing
          n214 = Unbundle By Name(w565) -> ("Channel Properties.Channel Name"=w564:string)
          n215 = call "Split_Ch_name.vi"("Ch name"=w564) -> ("Low level"=w562:string)  [unwired: 2 out]
          n216 = Format Into String(format string="%s=%.1f, " ("Format String"), w562, w558) -> (resulting string=w559:string)  [unwired: 2 in, 1 out]
          n217 = Concatenate Strings(w563, w559) -> (w560:string)
        }
        n218 = case shown="\"Move traverse\"" w541 {
          tunnel: ["When requesting a move." "When reading position." "When teaching position."] -> w540
          frame "Move traverse" {
          }
          frame "Read traverse position" {
          }
          frame "Teach Position" {
          }
        }
        n219 = Concatenate Strings(w544, w543, w540) -> (w542:string)
      }
    }
  }
  "Error String" <- w7
